vi "Close Client Context.vi"(8 "error in (no error)":errorcluster, 11 "ContextID":T1) -> (0 "error out":errorcluster)   [LabVIEW 2019, in "grpc-lvsupport.lvlib"]
uses:
  grpc-lvsupport.lvlib
  grpcId.ctl
  <vilib>/Utility/error.llb/Error Cluster From Error Code.vi
  <resource>/labview_grpc_server.dll
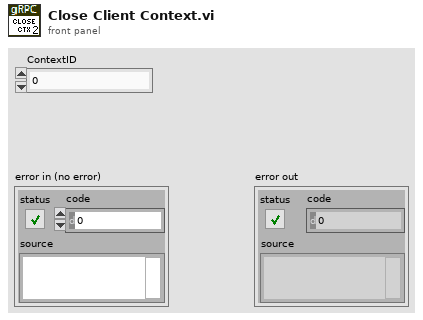
[diagram p1: front panel]
types:
  T1 = typedef "grpc-lvsupport.lvlib/grpcId.ctl" = u64
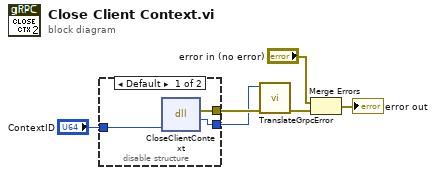
[diagram p0: block diagram]
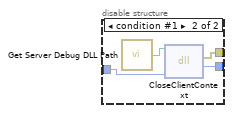
[diagram p2: hidden frame]
diagram:
  n1 = disable-structure shown="Default" {
    disable-tunnel: [w9 w13] -> w6
    disable-tunnel: [w8 w11] -> w5
    disable-tunnel: "ContextID" -> [w7 w10]
    frame condition #0 (active) {
      n2 = dll-call lib="C:/Program Files (x86)/National Instruments/LabVIEW 2024/resource/labview_grpc_server.*" fn="CloseClientContext"("contextId"=w7) -> (error out=w9:errorcluster, "return type"=w8:i32)  [unwired: 4 in, 1 out]
    }
    frame condition #1 {
      n3 = call "Get Server Debug DLL Path.vi"() -> ("DLL Path"=w12:path)
      n4 = dll-call lib="?" fn="CloseClientContext"(path in=w12, "contextId"=w10) -> (error out=w13:errorcluster, "return type"=w11:i32)  [unwired: 3 in, 1 out]
    }
  }
  n5 = call "TranslateGrpcError.vi"("error in"=w6, "Error Code"=w5) -> ("error out"=w4:errorcluster)  [unwired: 9 in]
  n6 = Merge Errors("error in (no error)", w4) -> (→"error out":errorcluster)
